vi "PC main4.vi"() -> ()   [LabVIEW 2019]
panel:
  out "Numeric 3":i32
  out "Last J 2":dbl
  out "State":i16
  in  "PD Time[s]":dbl
  in  "Individual Time[s]":dbl
  in  "stop":bool
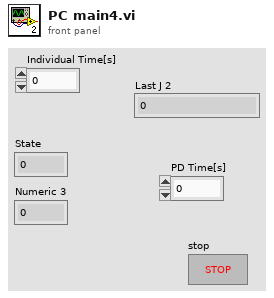
[diagram p1: front panel]
types:
  T1 = enum16{"open", "replace", "create", "open or create", "replace or create", "replace or create with confirmation"}
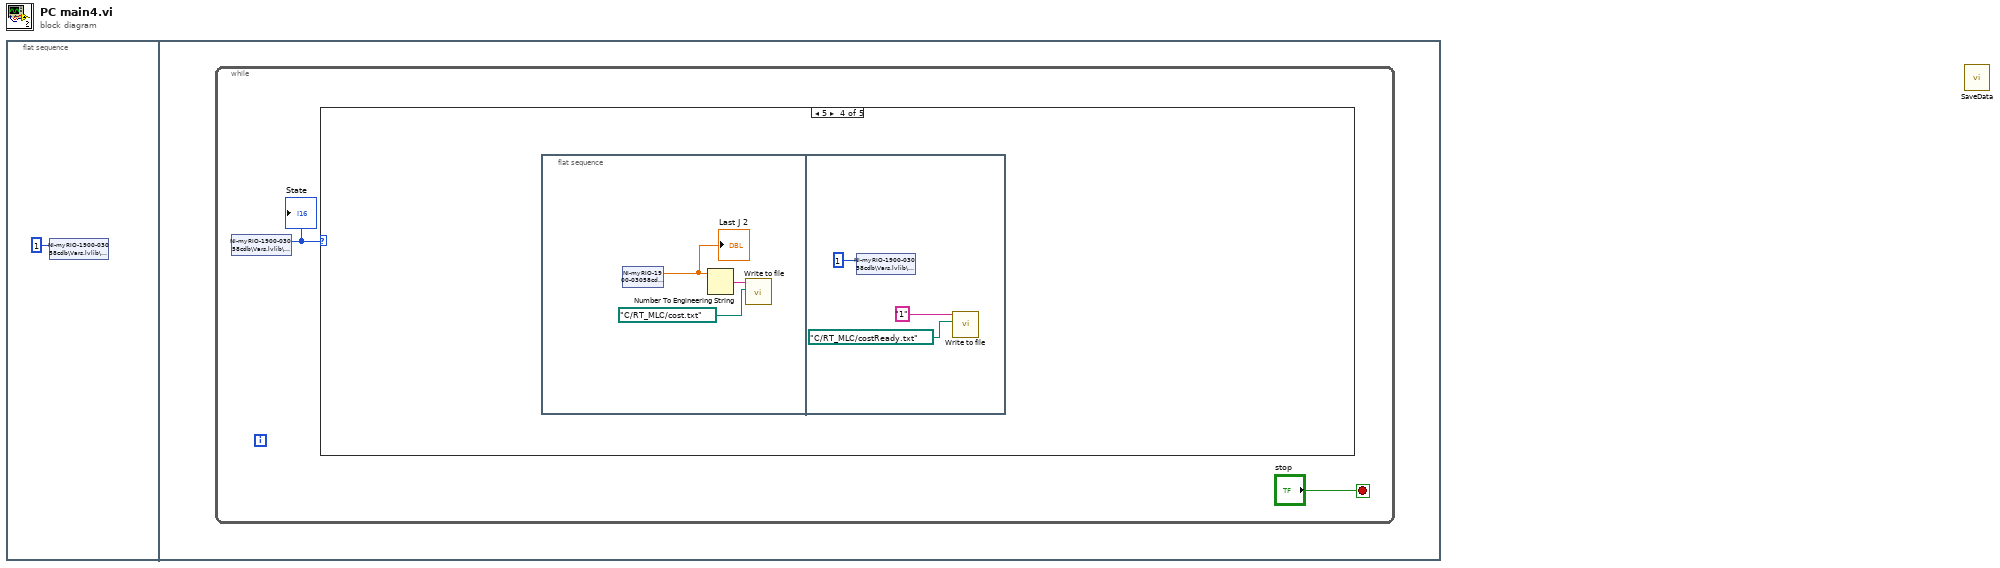
[diagram p0: block diagram]
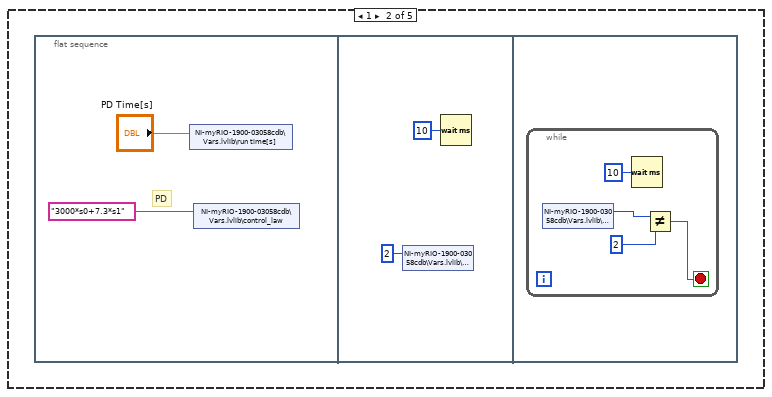
[diagram p3: hidden frame]
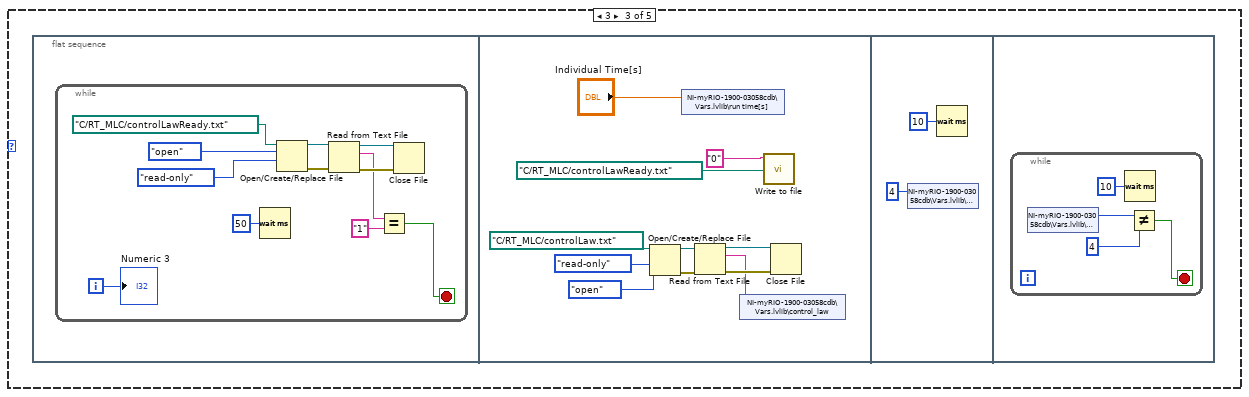
[diagram p4: hidden frame]
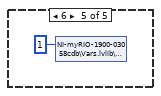
[diagram p5: hidden frame]
diagram:
  n1 = flat-sequence {
    frame #0 {
      n2 = shared-variable "NI-myRIO-1900-03058cdb\\Vars.lvlib\\State"(i16 1 ("State")) -> ()  [unwired: 1 in, 1 out]
    }
    frame #1 {
      n3 = while "Timed Loop" {
        stop <- "stop" stop-if-true
        n4 = shared-variable "NI-myRIO-1900-03058cdb\\Vars.lvlib\\State"() -> (w2:i16)  [unwired: 1 in, 1 out]
        "State" <- w2
        n5 = case shown="5" w2 {
          frame Default {
          }
          frame 1 {
            n6 = flat-sequence {
              frame #0 {
                # "PD"
                n7 = shared-variable "NI-myRIO-1900-03058cdb\\Vars.lvlib\\run time[s]"("PD Time[s]") -> ()  [unwired: 1 in, 1 out]
                n8 = shared-variable "NI-myRIO-1900-03058cdb\\Vars.lvlib\\control_law"("3000*s0+7.3*s1") -> ()  [unwired: 1 in, 1 out]
              }
              frame #1 {
                n9 = shared-variable "NI-myRIO-1900-03058cdb\\Vars.lvlib\\State"(i16 2 ("State")) -> ()  [unwired: 1 in, 1 out]
                n10 = Wait (ms)(milliseconds to wait=u32 10) -> ()  [unwired: 1 out]
              }
              frame #2 {
                n11 = while {
                  stop <- w9 stop-if-true
                  n12 = shared-variable "NI-myRIO-1900-03058cdb\\Vars.lvlib\\State"() -> (w11:i16)  [unwired: 1 in, 1 out]
                  n13 = Wait (ms)(milliseconds to wait=u32 10) -> ()  [unwired: 1 out]
                  n14 = Not Equal?(x=w11, y=i16 2) -> (x != y?=w9:bool)
                }
              }
            }
          }
          frame 3 {
            n15 = flat-sequence {
              frame #0 {
                n16 = while {
                  i -> [w13]
                  stop <- w12 stop-if-true
                  n17 = Wait (ms)(milliseconds to wait=u32 50) -> ()  [unwired: 1 out]
                  n18 = Open/Create/Replace File(file path (use dialog)=path "C:/RT_MLC/controlLawReady.txt", operation (0:open)=T1."open", access (0:read/write)=enum16{"read/write", "read-only", "write-only"}."read-only") -> (refnum out=w19:refnum<file>, error out=w20:errorcluster)  [unwired: 3 in, 1 out]
                  n19 = Read from Text File(file (use dialog)=w19, error in=w20) -> (refnum out=w21:refnum<file>, text=w14:string, error out=w22:errorcluster)  [unwired: 2 in, 1 out]
                  n20 = Equal?(x=w14, y="1") -> (x = y?=w12:bool)
                  n21 = Close File(refnum=w21, error in=w22) -> ()  [unwired: 2 out]
                  "Numeric 3" <- w13
                }
              }
              frame #1 {
                n22 = Open/Create/Replace File(file path (use dialog)=path "C:/RT_MLC/controlLaw.txt", operation (0:open)=T1."open", access (0:read/write)=enum16{"read/write", "read-only", "write-only"}."read-only") -> (refnum out=w33:refnum<file>, error out=w34:errorcluster)  [unwired: 3 in, 1 out]
                n23 = shared-variable "NI-myRIO-1900-03058cdb\\Vars.lvlib\\run time[s]"("Individual Time[s]") -> ()  [unwired: 1 in, 1 out]
                n24 = Read from Text File(file (use dialog)=w33, error in=w34) -> (refnum out=w28:refnum<file>, text=w27:string, error out=w29:errorcluster)  [unwired: 2 in, 1 out]
                n25 = shared-variable "NI-myRIO-1900-03058cdb\\Vars.lvlib\\control_law"(w27) -> ()  [unwired: 1 in, 1 out]
                n26 = call "Write to file.vi"("file path (use dialog)"=path "C:/RT_MLC/controlLawReady.txt", "String"="0" ("text")) -> ()  [unwired: 10 in]
                n27 = Close File(refnum=w28, error in=w29) -> ()  [unwired: 2 out]
              }
              frame #2 {
                n28 = shared-variable "NI-myRIO-1900-03058cdb\\Vars.lvlib\\State"(i16 4 ("State")) -> ()  [unwired: 1 in, 1 out]
                n29 = Wait (ms)(milliseconds to wait=u32 10) -> ()  [unwired: 1 out]
              }
              frame #3 {
                n30 = while {
                  stop <- w38 stop-if-true
                  n31 = shared-variable "NI-myRIO-1900-03058cdb\\Vars.lvlib\\State"() -> (w40:i16)  [unwired: 1 in, 1 out]
                  n32 = Wait (ms)(milliseconds to wait=u32 10) -> ()  [unwired: 1 out]
                  n33 = Not Equal?(x=w40, y=i16 4) -> (x != y?=w38:bool)
                }
              }
            }
          }
          frame 5 {
            n34 = flat-sequence {
              frame #0 {
                n35 = shared-variable "NI-myRIO-1900-03058cdb\\Vars.lvlib\\J"() -> (w42:dbl)  [unwired: 1 in, 1 out]
                "Last J 2" <- w42
                n36 = Number To Engineering String(4:w42) -> (0:w41:string)  [unwired: 3 in]
                n37 = call "Write to file.vi"("file path (use dialog)"=path "C:/RT_MLC/cost.txt", "String"=w41) -> ()  [unwired: 10 in]
              }
              frame #1 {
                n38 = shared-variable "NI-myRIO-1900-03058cdb\\Vars.lvlib\\State"(i16 1 ("State")) -> ()  [unwired: 1 in, 1 out]
                n39 = call "Write to file.vi"("file path (use dialog)"=path "C:/RT_MLC/costReady.txt", "String"="1" ("text")) -> ()  [unwired: 10 in]
              }
            }
          }
          frame 6 {
            n40 = shared-variable "NI-myRIO-1900-03058cdb\\Vars.lvlib\\State"(i16 1 ("State")) -> ()  [unwired: 1 in, 1 out]
          }
        }
      }
    }
  }
  n41 = call "SaveData.vi"() -> ()  [unwired: 12 in]
